vi "TCP-VISA_omega.vi"() -> ()   [LabVIEW 2016]
panel:
  out "Read errors":i32
  out "code":i32
  out "Waveform Chart":dbl(graph)
  out "Oven Temperature":dbl
  in  "VISA resource name":refnum<visa-resource-name>="TCPIP0::192.168.1.160::966::SOCKET"
  in  "byte count":u32=15
  out "Iteration":i32
  in  "Wait (ms)":u32=500
  in  "stop":bool
  out "read buffer":string
  out "error out":errorcluster
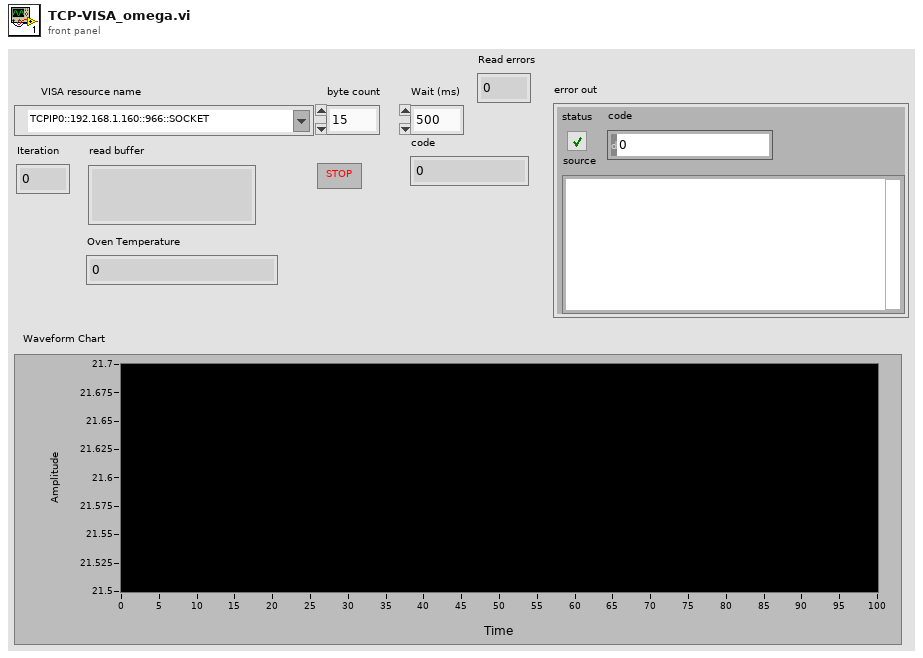
[diagram p1: front panel]
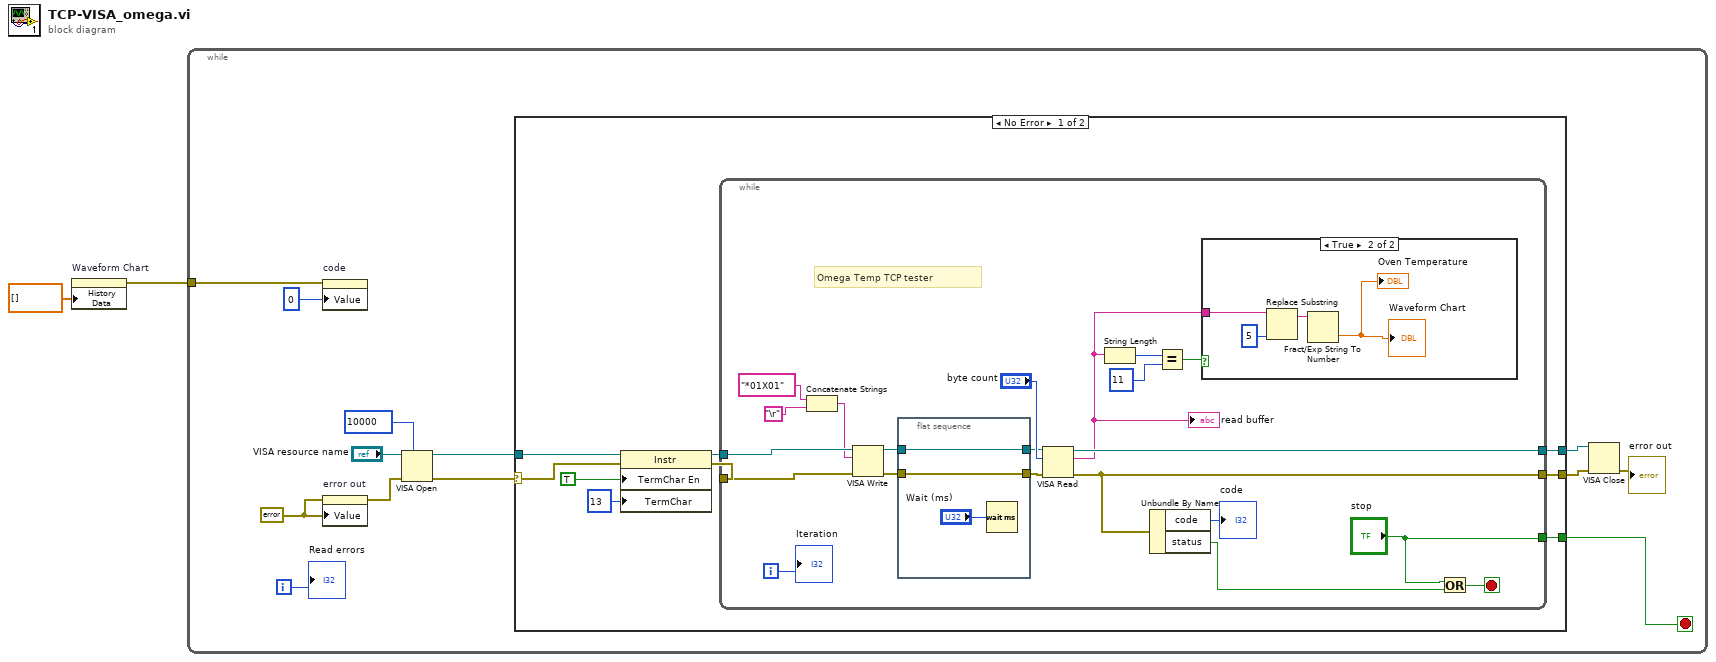
[diagram p0: block diagram]
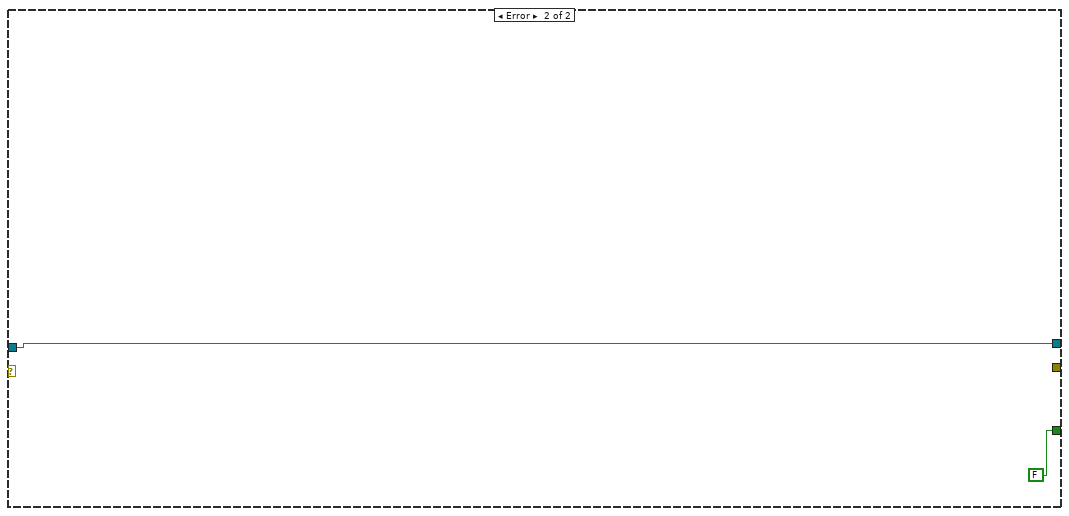
[diagram p3: hidden frame]
diagram:
  n1 = property on="Waveform Chart" class="WFChart (strict)"("History Data"=dbl[] []) -> (error out=w1:errorcluster)  [unwired: 2 in, 1 out]
  n2 = while {
    tunnel: w1 -> [w4]
    i -> [w5]
    stop <- w6 stop-if-true
    w8 = errorcluster {"status"=FALSE, "code"=0, "source"=""} ("error in (no error)")
    n3 = property on="code" class="DigNum (strict)"(error in=w4, "Value"=0 ("code")) -> ()  [unwired: 1 in, 2 out]
    n4 = property on="error out" class="Clust (strict)"(error in=w8, "Value"=w8) -> (error out=w10:errorcluster)  [unwired: 1 in, 1 out]
    n5 = VISA Open(timeout (0)=u32 10000 ("VISA Open timeout (0)"), error in (no error)=w10, VISA resource name="VISA resource name") -> (VISA resource name=w15:refnum<visa-resource-name>, error out=w11:errorcluster)  [unwired: 2 in]
    n6 = case shown="No Error" w11 {
      selector: w11 -> [w16 _]
      tunnel: w15 -> [w22 w54]
      tunnel: [w24 w54] -> w14
      tunnel: [w23 w55] -> w13
      tunnel: [w17 FALSE ("stop")] -> w6
      frame No Error {
        n7 = property class="Instr"(reference=w22, error in=w16, "TermChar En"=TRUE ("Message Based Settings:Termination Character Enable"), "TermChar"=u8 13 ("Message Based Settings:Termination Character")) -> (reference out=w21:refnum<visa-resource-name>, error out=w20:errorcluster)
        n8 = while {
          tunnel: w21 -> [w41]
          tunnel: [w45] -> w24
          tunnel: w20 -> [w36]
          tunnel: [w44] -> w23
          tunnel: ["stop"] -> w17
          i -> [w42]
          stop <- w43 stop-if-true
          # "Omega Temp TCP tester"
          n9 = Concatenate Strings("*01X01" ("data in"), "\r") -> (w38:string)
          n10 = VISA Write(VISA resource name=w41, write buffer=w38, error in (no error)=w36) -> (VISA resource name out=w28:refnum<visa-resource-name>, error out=w30:errorcluster)  [unwired: 1 out]
          n11 = flat-sequence {
            tunnel: w30 -> [w48]
            tunnel: [w48] -> w29
            tunnel: w28 -> [w47]
            tunnel: [w47] -> w27
            frame #0 {
              n12 = Wait (ms)(milliseconds to wait="Wait (ms)") -> ()  [unwired: 1 out]
            }
          }
          n13 = VISA Read(VISA resource name=w27, byte count="byte count", error in (no error)=w29) -> (VISA resource name out=w45:refnum<visa-resource-name>, read buffer=w32:string, error out=w44:errorcluster)  [unwired: 1 out]
          "read buffer" <- w32
          n14 = String Length(string=w32) -> (length=w35:i32)
          n15 = Unbundle By Name(w44) -> ("code"=→"code":i32, "status"=w26:bool)
          n16 = Equal?(x=w35, y=11) -> (x = y?=w33:bool)
          n17 = case shown="True" w33 {
            tunnel: w32 -> [_ w49]
            frame False {
            }
            frame True {
              n18 = Replace Substring(2:5 ("length (len. of substring)"), 5:w49) -> (1:w50:string)  [unwired: 2 in, 1 out]
              n19 = Fract/Exp String To Number(string=w50) -> (number=→"Oven Temperature" →"Waveform Chart":dbl)  [unwired: 3 in, 1 out]
            }
          }
          n20 = Or(x="stop", y=w26) -> (x .or. y?=w43:bool)
          "Iteration" <- w42
        }
      }
      frame Error {
      }
    }
    n21 = VISA Close(VISA resource name=w14, error in (no error)=w13) -> (error out=→"error out":errorcluster)
    "Read errors" <- w5
  }
